vi "Create Channel Task.vi"(5 "Duty cycle":dbl=0.5 format="%.6f", 7 "Frequency":dbl=1.0 format="%.6f", 8 "error in":errorcluster, 10 "SQL query":string="SELECT max(Frequency),max(DutyCycle), max(SampleRate) FROM ltt.daq_configuration \nWhere ChannelType='PWM_Output' and Enabled=1;", 11 "NI PWM Output in":refnum<class "NI PWM Output.lvclass">) -> (0 "error out":errorcluster, 3 "NI PWM Output out":refnum<class "NI PWM Output.lvclass">)   [LabVIEW 2023, in "HardwareAbstractionLayer_LVOOP.lvlib" / "NI PWM Output.lvclass"]
doc: "This VI Analog Output Physical Channel Based DAQmx Create Channel"
uses:
  NI PWM Output.lvclass
  NI PWM Output.lvclass/NI PWM Output.ctl
  <vilib>/DAQmx/create/channels.llb/DAQmx Create Channel (CO-Pulse Generation-Frequency).vi
  <vilib>/DAQmx/configure/timing.llb/DAQmx Timing (Implicit).vi
  <resource>/objmgr/daqmx.rc
  Teststand/Teststand.lvclass
panel:
  out "CO Pulse Duty Cycle":dbl[](array[numeric])
  out "CO Pulse Frequency":dbl[](array[numeric])
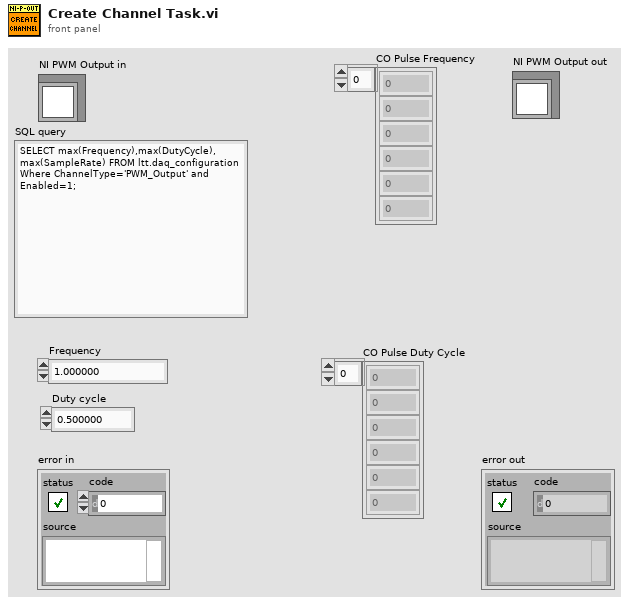
[diagram p1: front panel]
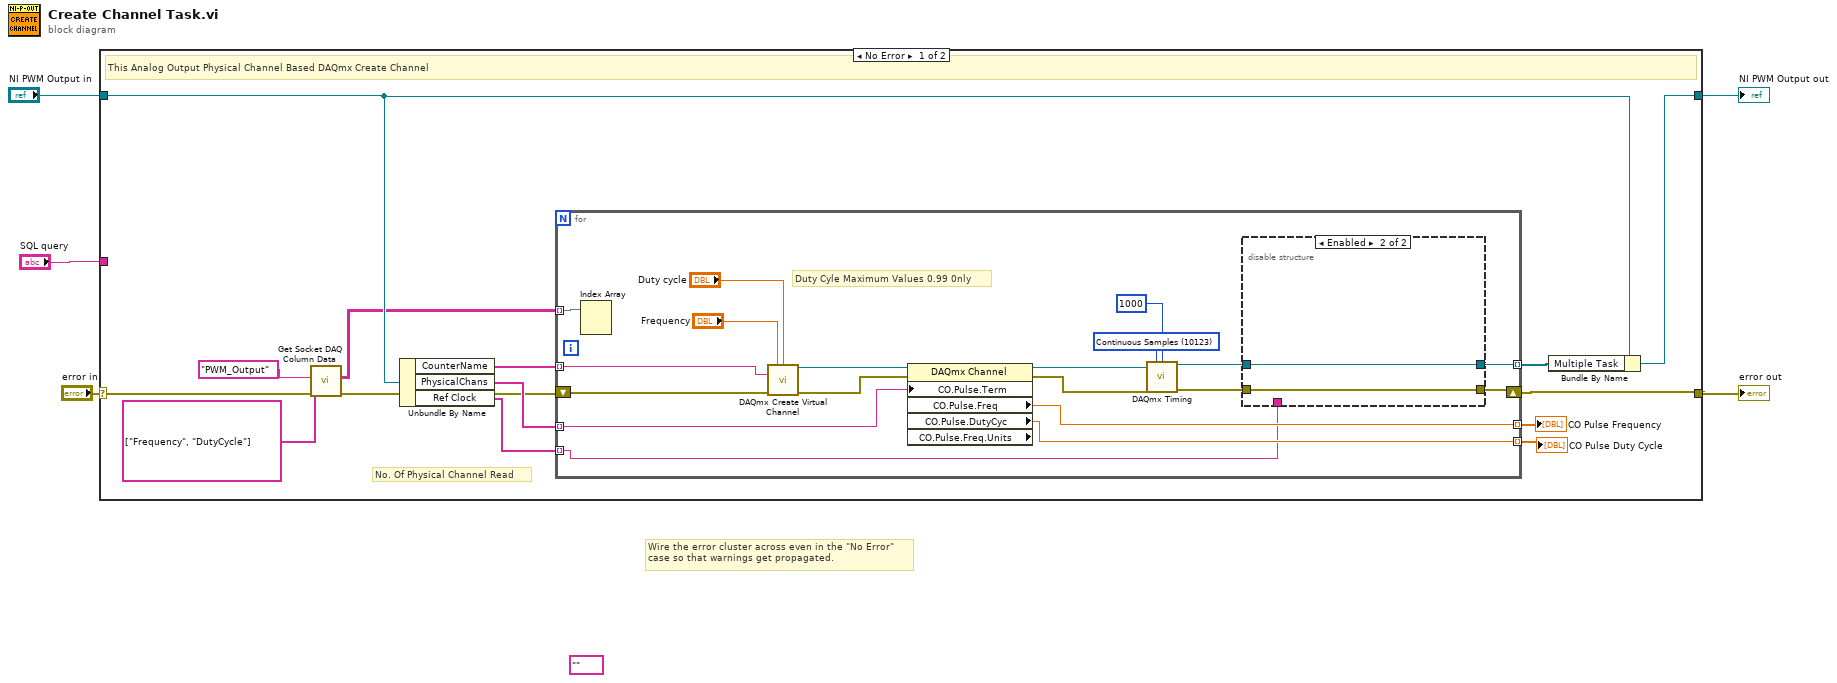
[diagram p0: block diagram]
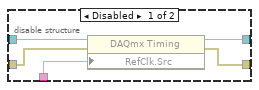
[diagram p2: hidden frame]
diagram:
  (unwired) tag ""
  # "Wire the error cluster across even in the \"No Error\"\ncase so that warnings get propagated."
  n1 = case shown="No Error" "error in" {
    selector: "error in" -> [w11 w47]
    tunnel: [w12 w47] -> w4
    tunnel: [w19 w46] -> w2
    tunnel: "NI PWM Output in" -> [w18 w46]
    tunnel: "SQL query" -> [_ _]
    frame No Error {
      # "No. Of Physical Channel Read"
      # "This Analog Output Physical Channel Based DAQmx Create Channel"
      n2 = call "Get Socket DAQ Column Data.vi"("error In"=w11, "columns"=string[] ["Frequency", "DutyCycle"], "ChannelType"="PWM_Output") -> ("error out"=w10:errorcluster, "Data"=w9:string[][])  [unwired: 7 in]
      n3 = Unbundle By Name(w18) -> ("CounterName"=w14:tag[], "PhysicalChans"=w17:tag[], "Ref Clock"=w6:tag[])
      n4 = for {
        tunnel: w14 -> [w37] mode=indexing
        tunnel: w17 -> [w34] mode=indexing
        shift-right: [w24] -> w12
        shift-left: w10 -> [w38]
        tunnel: [w33] -> w16 mode=indexing
        tunnel: [w32] -> w15 mode=indexing
        tunnel: [w25] -> w13 mode=indexing
        tunnel: w9 -> [w26] mode=indexing
        tunnel: w6 -> [w22] mode=indexing
        w31 = 10123 items=["Finite Samples"=10178, "Continuous Samples"=10123, "Hardware Timed Single Point"=12522] ("sample mode")
        # "Duty Cyle Maximum Values 0.99 0nly"
        n5 = Index Array(array=w26) -> ()  [unwired: 2 in, 2 out]
        n6 = call-poly <vilib>:"DAQmx Create Virtual Channel.vi"("frequency"="Frequency", "duty cycle"="Duty cycle", "counter"=w37, "error in"=w38) -> ("task out"=w36:refnum<k21>, "error out"=w35:errorcluster)  [unwired: 10 in]
        n7 = property class="DAQmx Channel" props=["CO.Pulse.Term", "CO.Pulse.Freq", "CO.Pulse.DutyCyc", "CO.Pulse.Freq.Units"](reference=w36, error in=w35, "CO.Pulse.Term"=w34) -> (reference out=w30:refnum<k21>, error out=w29:errorcluster, "CO.Pulse.Freq"=w33:dbl, "CO.Pulse.DutyCyc"=w32:dbl)  [unwired: 1 out]
        n8 = call-poly <vilib>:"DAQmx Timing.vi"("task/channels in"=w30, "sample mode"=w31, "samples per channel"=1000, "error in"=w29) -> ("task out"=w28:refnum<k21>, "error out"=w27:errorcluster)  [unwired: 10 in]
        n9 = disable-structure shown="Enabled" {
          disable-tunnel: w28 -> [w43 w45]
          disable-tunnel: w27 -> [w42 w44]
          disable-tunnel: [w40 w45] -> w25
          disable-tunnel: [w41 w44] -> w24
          disable-tunnel: w22 -> [w39 _]
          frame Disabled {
            n10 = property class="DAQmx Timing"(reference=w43, error in=w42, "RefClk.Src"=w39) -> (reference out=w40:refnum<k21>, error out=w41:errorcluster)
          }
          frame Enabled {
          }
        }
      }
      "CO Pulse Frequency" <- w16
      "CO Pulse Duty Cycle" <- w15
      n11 = Bundle By Name(cluster=w18, "Multiple Task"=w13) -> (w19:refnum<class "NI PWM Output.lvclass">)
    }
    frame Error {
    }
  }
  "error out" <- w4
  "NI PWM Output out" <- w2
